vi "Generate_WayPoints_Hopping_IT_away_from_Surface.vi"(11 "Input Cluster":T2={"Scan Rate (um/s)"=15.0, "X Start"=15.0, "X End"=15.0, "Y Start"=15.0, "Y End"=15.0, " Z Start"=15.0, "HoppingDistance"=1.0, "V"=15.0, "Z End"=15.0, "Approach Rate Hopping (um/s)"=15.0, "V_i-t"=15.0, "HoldTime Bulk Pre IT/s "=15.0, "HoldTime Bulk IT /s"=15.0, "Retrack Rate to away from surface (um/s)"=0.005, "Retrack Rate to bulk (um/s) "=1.0}) -> (0 "output cluster":T1)   [LabVIEW 2023]
uses:
  TypeDefs/WayPointCluster.ctl
panel:
  in  "WayPointCluster":T1
  out "Y  P":dbl
  out "X  P":dbl
  out "HoppingDistanceX":dbl
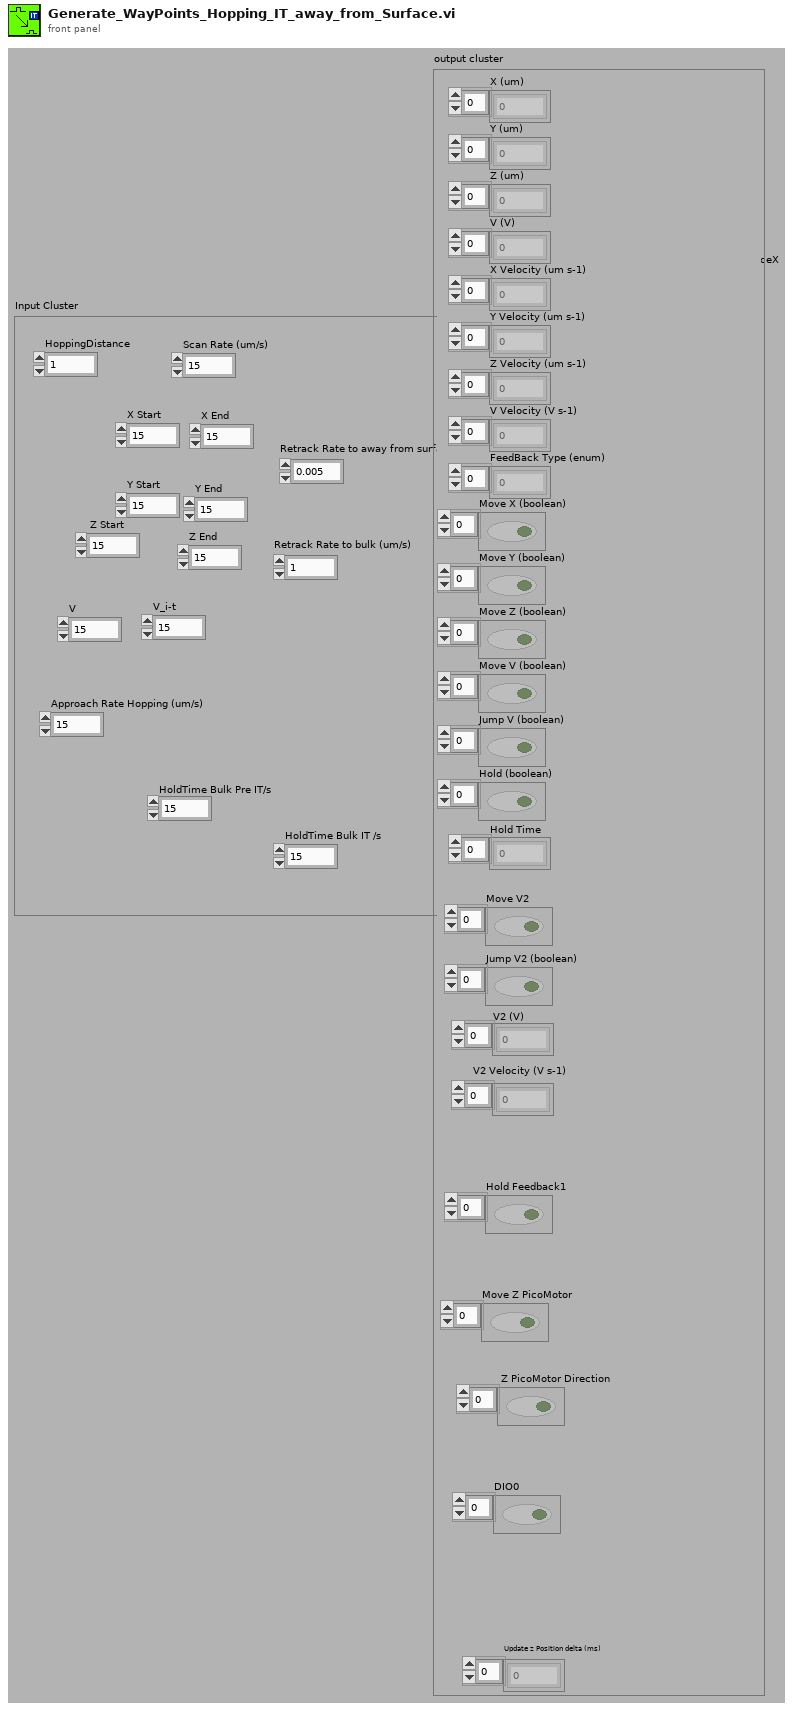
[diagram p1: front panel]
types:
  T1 = typedef "WayPointCluster.ctl" = cluster{"X (um)":dbl[], "Y (um)":dbl[], "Z (um)":dbl[], "V (V)":dbl[], "X Velocity (um s-1)":dbl[], "Y Velocity (um s-1)":dbl[], "Z Velocity (um s-1)":dbl[], "V Velocity (V s-1)":dbl[], "FeedBack Type (enum)":u16[], "Move X (boolean)":bool[], "Move Y (boolean)":bool[], "Move Z (boolean)":bool[], "Move V (boolean)":bool[], "Jump V (boolean)":bool[], "Hold (boolean)":bool[], "Hold Time":u32[], "V2 (V)":dbl[], "Move V2":bool[], "V2 Velocity (V s-1)":dbl[], "Jump V2 (boolean)":bool[], "Update z Position delta (ms)":i16[], "Hold Feedback1":bool[], "Move Z PicoMotor":bool[], " Z PicoMotor Direction":bool[], "DIO0":bool[]}
  T2 = cluster{"Scan Rate (um/s)":dbl, "X Start":dbl, "X End":dbl, "Y Start":dbl, "Y End":dbl, " Z Start":dbl, "HoppingDistance":dbl, "V":dbl, "Z End":dbl, "Approach Rate Hopping (um/s)":dbl, "V_i-t":dbl, "HoldTime Bulk Pre IT/s ":dbl, "HoldTime Bulk IT /s":dbl, "Retrack Rate to away from surface (um/s)":dbl, "Retrack Rate to bulk (um/s) ":dbl}
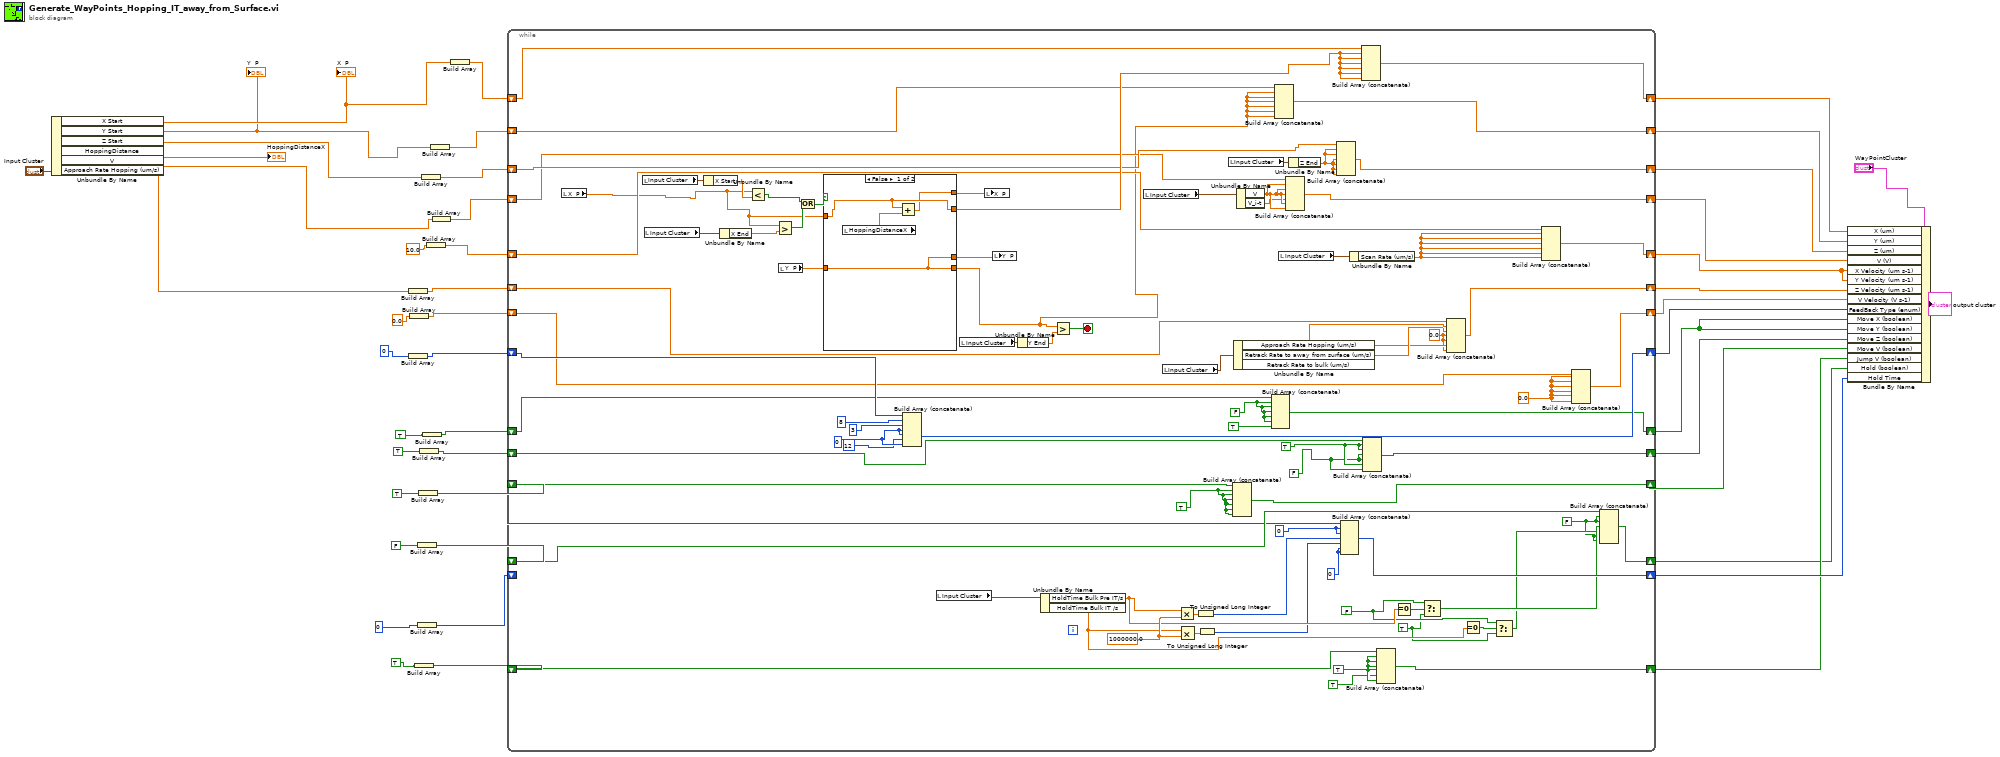
[diagram p0: block diagram]
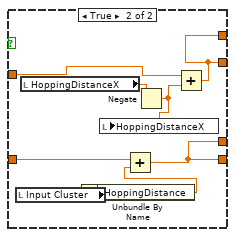
[diagram p2: hidden frame]
diagram:
  n1 = Unbundle By Name("Input Cluster") -> ("X Start"=w28:dbl, "Y Start"=w27:dbl, "Z Start"=w29:dbl, "HoppingDistance"=→"HoppingDistanceX":dbl, "V"=w26:dbl, "Approach Rate Hopping (um/s)"=w11:dbl)
  "X  P" <- w28
  "Y  P" <- w27
  n2 = Build Array(w11) -> (w36:dbl[])
  n3 = Build Array(u16 0 ("element")) -> (w32:u16[])
  n4 = Build Array(0.0 ("element")) -> (w34:dbl[])
  n5 = Build Array(TRUE) -> (w21:bool[])
  n6 = Build Array(FALSE) -> (w14:bool[])
  n7 = Build Array(u32 0 ("element")) -> (w24:u32[])
  n8 = Build Array(TRUE) -> (w19:bool[])
  n9 = Build Array(TRUE) -> (w25:bool[])
  n10 = Build Array(w29) -> (w41:dbl[])
  n11 = Build Array(TRUE) -> (w2:bool[])
  n12 = Build Array(10.0 ("element")) -> (w37:dbl[])
  n13 = Build Array(w27) -> (w43:dbl[])
  n14 = Build Array(w26) -> (w39:dbl[])
  n15 = Build Array(w28) -> (w45:dbl[])
  n16 = while {
    shift-right: [w114] -> w44
    shift-left: w45 -> [w66]
    shift-right: [w111] -> w42
    shift-left: w43 -> [w112]
    shift-right: [w109] -> w40
    shift-left: w41 -> [w110]
    shift-right: [w106] -> w38
    shift-left: w39 -> [w86]
    shift-right: [w105] -> w4
    shift-left: w37 -> [w107]
    shift-right: [w103] -> w35
    shift-left: w36 -> [w104]
    shift-right: [w101] -> w33
    shift-left: w34 -> [w102]
    shift-right: [w128] -> w31
    shift-left: w32 -> [w129]
    shift-right: [w99] -> w23
    shift-left: w25 -> [w100]
    shift-right: [w94] -> w7
    shift-left: w14 -> [w95]
    shift-right: [w92] -> w22
    shift-left: w24 -> [w93]
    shift-right: [w89] -> w20
    shift-left: w21 -> [w90]
    shift-right: [w97] -> w6
    shift-left: w19 -> [w98]
    shift-right: [w76] -> w1
    shift-left: w2 -> [w78]
    stop <- w83 stop-if-true
    w67 = TRUE
    w68 = FALSE
    w60 = u32 0 ("element")
    w77 = FALSE
    w79 = 0.0 ("element")
    w75 = 1000000.0 ("element")
    w88 = TRUE
    w96 = TRUE
    w64 = u32 0 ("element")
    w54 = FALSE
    w57 = FALSE
    w58 = TRUE
    w61 = u16 0 ("element")
    w49 = 0.0 ("element")
    n17 = local read "X  P"() -> (w84:dbl)
    n18 = local read "Input Cluster"() -> (w131:T2)
    n19 = local read "Input Cluster"() -> (w130:T2)
    n20 = Unbundle By Name(w131) -> ("X Start"=w125:dbl)
    n21 = Unbundle By Name(w130) -> ("X End"=w123:dbl)
    n22 = Less?(x=w84, y=w125) -> (x < y?=w124:bool)
    n23 = Greater?(x=w84, y=w123) -> (0:w122:bool)
    n24 = local read "Y  P"() -> (w118:dbl)
    n25 = Or(x=w124, y=w122) -> (x .or. y?=w121:bool)
    n26 = case shown="False" w121 {
      tunnel: [w133 w136] -> w113
      tunnel: w84 -> [w133 w137]
      tunnel: w118 -> [w135 w140]
      tunnel: [w135 w139] -> w82
      tunnel: [w135 w139] -> w117
      tunnel: [w132 w136] -> w116
      frame False {
        n27 = local read "HoppingDistanceX"() -> (w134:dbl)
        n28 = Add(x=w133, y=w134) -> (x+y=w132:dbl)
      }
      frame True {
        n29 = local read "Input Cluster"() -> (w142:T2)
        n30 = local read "HoppingDistanceX"() -> (w143:dbl)
        n31 = Unbundle By Name(w142) -> ("HoppingDistance"=w141:dbl)
        n32 = Add(x=w140, y=w141) -> (x+y=w139:dbl)
        n33 = Negate(x=w143) -> (-x=w138:dbl)
        n34 = local write "HoppingDistanceX"(w138) -> ()
        n35 = Add(x=w137, y=w138) -> (x+y=w136:dbl)
      }
    }
    n36 = Build Array (concatenate)(w129, u16 8 ("element"), u16 3 ("element"), w61, w61, u16 12 ("element"), w61) -> (w128:u16[])
    n37 = local read "Input Cluster"() -> (w91:T2)
    n38 = local read "Input Cluster"() -> (w120:T2)
    n39 = local write "X  P"(w116) -> ()
    n40 = local write "Y  P"(w117) -> ()
    n41 = Unbundle By Name(w120) -> ("Y End"=w119:dbl)
    n42 = Unbundle By Name(w91) -> ("HoldTime Bulk Pre IT/s"=w72:dbl, "HoldTime Bulk IT /s"=w71:dbl)
    n43 = Greater?(x=w82, y=w119) -> (0:w83:bool)
    n44 = local read "Input Cluster"() -> (w126:T2)
    n45 = local read "Input Cluster"() -> (w115:T2)
    n46 = Multiply(x=w72, y=w75) -> (x*y=w74:dbl)
    n47 = Multiply(x=w71, y=w75) -> (x*y=w73:dbl)
    n48 = To Unsigned Long Integer(number=w74) -> (unsigned 32bit integer=w63:u32)
    n49 = To Unsigned Long Integer(number=w73) -> (unsigned 32bit integer=w62:u32)
    n50 = local read "Input Cluster"() -> (w127:T2)
    n51 = Build Array (concatenate)(w98, w96, w96, w96, w96, w96, w96) -> (w97:bool[])
    n52 = Unbundle By Name(w115) -> ("Approach Rate Hopping (um/s)"=w52:dbl, "Retrack Rate to away from surface (um/s)"=w51:dbl, "Retrack Rate to bulk (um/s)"=w50:dbl)
    n53 = Unbundle By Name(w126) -> ("V"=w48:dbl, "V_i-t"=w47:dbl)
    n54 = Build Array (concatenate)(w78, w77, w77, w77, w77, w77, TRUE) -> (w76:bool[])
    n55 = Build Array (concatenate)(w112, w82, w82, w82, w82, w82, w82) -> (w111:dbl[])
    n56 = local read "Input Cluster"() -> (w85:T2)
    n57 = Build Array (concatenate)(w86, w48, w48, w48, w47, w48, w48) -> (w106:dbl[])
    n58 = Unbundle By Name(w127) -> ("Z End"=w108:dbl)
    n59 = Build Array (concatenate)(w110, w108, w108, w108, w108, w108, w108) -> (w109:dbl[])
    n60 = Build Array (concatenate)(w93, w64, w64, w63, w62, w60, w60) -> (w92:u32[])
    n61 = Unbundle By Name(w85) -> ("Scan Rate (um/s)"=w80:dbl)
    n62 = Build Array (concatenate)(w66, w113, w113, w113, w113, w113, w113) -> (w114:dbl[])
    n63 = Build Array (concatenate)(w100, w58, w58, w57, w57, w58, w57) -> (w99:bool[])
    n64 = Build Array (concatenate)(w90, w88, w88, w88, w88, TRUE, w88) -> (w89:bool[])
    n65 = Equal To 0?(x=w72) -> (x = 0?=w69:bool)
    n66 = Select(t=w68, s=w69, f=w67) -> (s? t:f=w56:bool)
    n67 = Build Array (concatenate)(w104, w52, w51, w49, w49, w50, w49) -> (w103:dbl[])
    n68 = Equal To 0?(x=w71) -> (x = 0?=w70:bool)
    n69 = Select(t=w68, s=w70, f=w67) -> (s? t:f=w55:bool)
    n70 = Build Array (concatenate)(w107, w80, w80, w80, w80, w80, w80) -> (w105:dbl[])
    n71 = Build Array (concatenate)(w102, w79, w79, w79, w79, w79, w79) -> (w101:dbl[])
    n72 = Build Array (concatenate)(w95, w54, w54, w56, w55, w54, w54) -> (w94:bool[])
  }
  n73 = Bundle By Name(cluster="WayPointCluster", "X (um)"=w44, "Y (um)"=w42, "Z (um)"=w40, "V (V)"=w38, "X Velocity (um s-1)"=w4, "Y Velocity (um s-1)"=w4, "Z Velocity (um s-1)"=w35, "V Velocity (V s-1)"=w33, "FeedBack Type (enum)"=w31, "Move X (boolean)"=w1, "Move Y (boolean)"=w1, "Move Z (boolean)"=w23, "Move V (boolean)"=w6, "Jump V (boolean)"=w20, "Hold (boolean)"=w7, "Hold Time"=w22) -> (→"output cluster":T1)
